vi "Configure Modulation (AM).vi"(0 "VISA resource name":refnum<visa-resource-name>, 1 "Enable AM (T: Enable)":bool=TRUE, 2 "Modulation Waveform (0: Sine)":u16(ring) items=["Sine", "Square", "Ramp", "Noise", "User Waveform", "Edit Memory", "EFile"], 5 "Channel (1: Channel 1)":u16(ring)=1 items=["Channel 1"=1, "Channel 2"=2], 7 "AM Source (0: Internal)":u16(ring) items=["Internal", "External"], 9 "Modulation Depth (3 %)":dbl=3.0, 11 "error in (no error)":errorcluster, 12 "Modulation Frequency (100 Hz)":dbl=100.0, 13 "User Waveform (0)":i32, 14 "EFile Name (\"\")":string) -> (4 "VISA resource name out":refnum<visa-resource-name>, 15 "error out":errorcluster)   [LabVIEW 2016, in "Tektronix AFG 1000 Series.lvlib"]
doc: "Configures and enables amplitude modulation (AM). In AM, the amplitude of the carrier is varied by the amplitude of the modulating waveform."
uses:
  Tektronix AFG 1000 Series.lvlib
panel:
  # "Internal AM Settings"
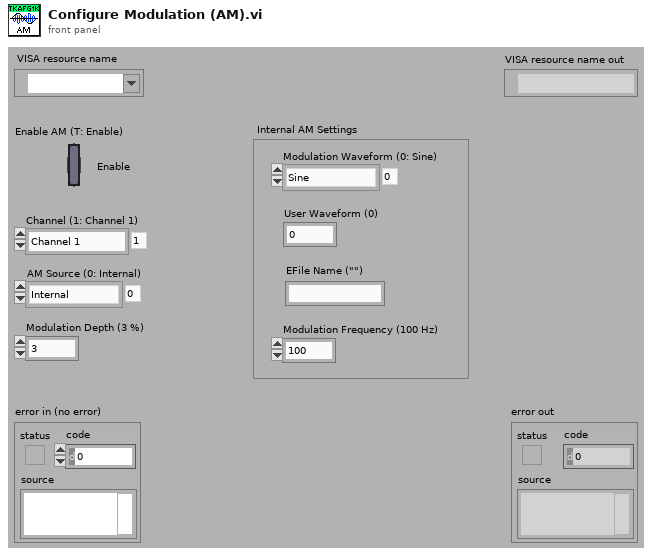
[diagram p1: front panel]
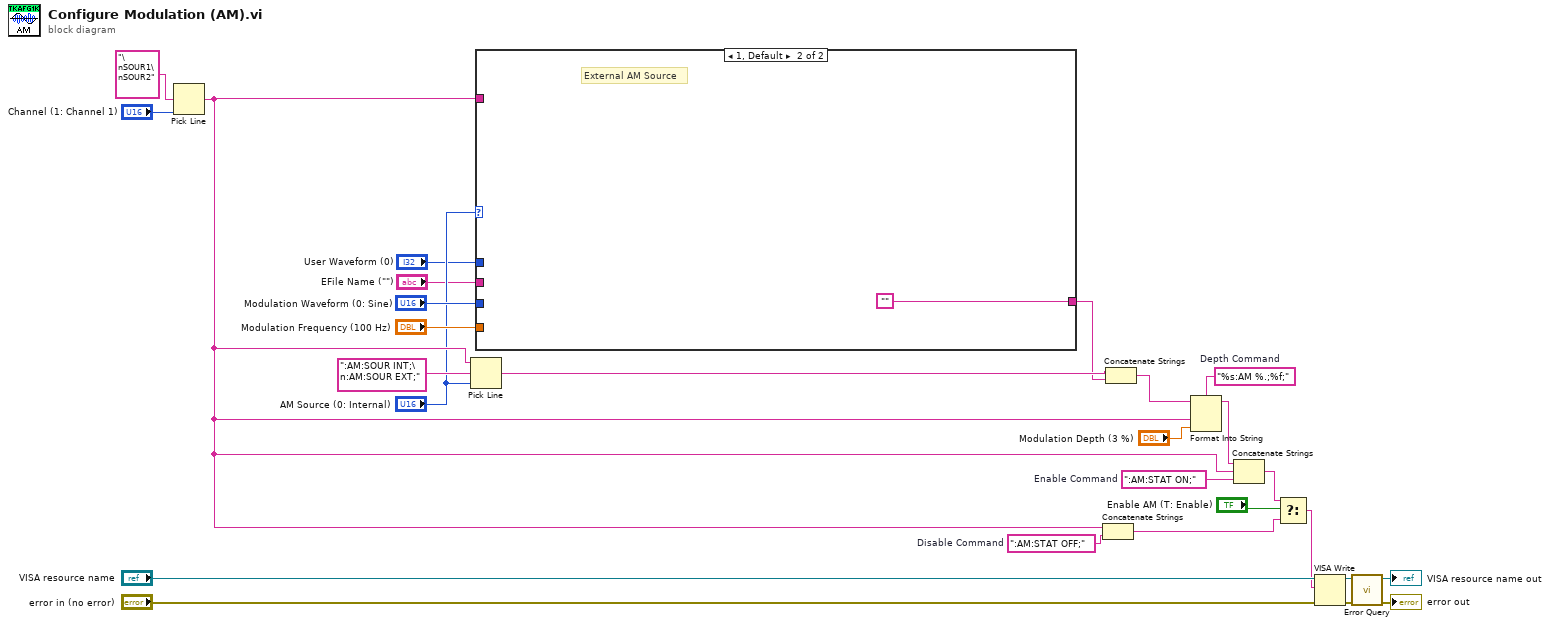
[diagram p0: block diagram]
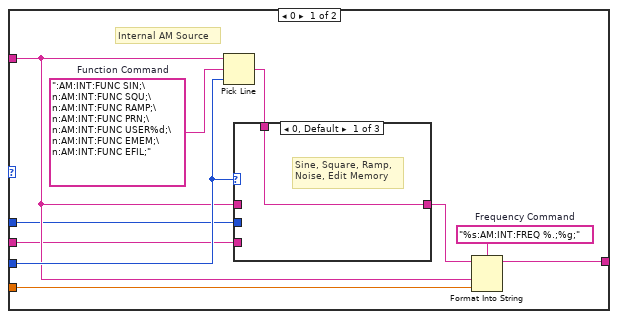
[diagram p2: hidden frame]
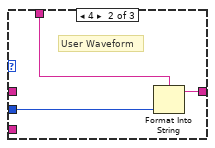
[diagram p3: hidden frame]
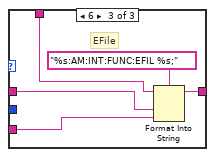
[diagram p4: hidden frame]
diagram:
  w18 = ":AM:STAT ON;"  # Enable Command
  w19 = "%s:AM %.;%f;"  # Depth Command
  w12 = ":AM:STAT OFF;"  # Disable Command
  n1 = Pick Line(multi-line string="\nSOUR1\nSOUR2" ("string (\"\")"), line index="Channel (1: Channel 1)") -> (output string=w4:string)  [unwired: 1 in]
  n2 = Pick Line(string ("")=w4, multi-line string=":AM:SOUR INT;\n:AM:SOUR EXT;" ("Source Command"), line index="AM Source (0: Internal)") -> (output string=w7:string)
  n3 = case shown="1, Default" "AM Source (0: Internal)" {
    tunnel: w4 -> [w30 _]
    tunnel: [w35 ""] -> w6
    tunnel: "Modulation Waveform (0: Sine)" -> [w31 _]
    tunnel: "Modulation Frequency (100 Hz)" -> [w34 _]
    tunnel: "User Waveform (0)" -> [w29 _]
    tunnel: "EFile Name (\"\")" -> [w28 _]
    frame 0 {
      w36 = "%s:AM:INT:FREQ %.;%g;"  # Frequency Command
      w37 = ":AM:INT:FUNC SIN;\n:AM:INT:FUNC SQU;\n:AM:INT:FUNC RAMP;\n:AM:INT:FUNC PRN;\n:AM:INT:FUNC USER%d;\n:AM:INT:FUNC EMEM;\n:AM:INT:FUNC EFIL;"  # Function Command
      # "Internal AM Source"
      n4 = Pick Line(string ("")=w30, multi-line string=w37, line index=w31) -> (output string=w33:string)
      n5 = case shown="0, Default" w31 {
        tunnel: w33 -> [w38 w41 w45]
        tunnel: [w38 w40 w46] -> w32
        tunnel: w30 -> [_ _ w43]
        tunnel: w29 -> [_ w39 _]
        tunnel: w28 -> [_ _ w42]
        frame 0, Default {
          # "Sine, Square, Ramp,\nNoise, Edit Memory"
        }
        frame 4 {
          # "User Waveform"
          n6 = Format Into String(format string=w41, w39) -> (resulting string=w40:string)  [unwired: 2 in, 1 out]
        }
        frame 6 {
          # "EFile"
          n7 = Format Into String(format string="%s:AM:INT:FUNC:EFIL %s;", initial string=w45, w43, w42) -> (resulting string=w46:string)  [unwired: 1 in, 1 out]
        }
      }
      n8 = Format Into String(format string=w36, initial string=w32, w30, w34) -> (resulting string=w35:string)  [unwired: 1 in, 1 out]
    }
    frame 1, Default {
      # "External AM Source"
    }
  }
  n9 = Concatenate Strings(w4, w12) -> (w11:string)
  n10 = Concatenate Strings(w7, w6) -> (w8:string)
  n11 = Format Into String(format string=w19, initial string=w8, w4, "Modulation Depth (3 %)") -> (resulting string=w5:string)  [unwired: 1 in, 1 out]
  n12 = Concatenate Strings(w5, w4, w18) -> (w14:string)
  n13 = Select(t=w14, s="Enable AM (T: Enable)", f=w11) -> (s? t:f=w15:string)
  n14 = VISA Write(VISA resource name="VISA resource name", write buffer=w15, error in (no error)="error in (no error)") -> (VISA resource name out=w23:refnum<visa-resource-name>, error out=w22:errorcluster)  [unwired: 1 out]
  n15 = call "Error Query.vi"("error in (no error)"=w22, "VISA resource name"=w23) -> ("error out"=→"error out":errorcluster, "VISA resource name out"=→"VISA resource name out":refnum<visa-resource-name>)  [unwired: 6 in, 2 out]
